vi "Read Pulse driver.vi"(8 "error in (no error)":errorcluster, 11 "Pulse Recorder in":refnum<class "Pulse Recorder Actor.lvclass">) -> (0 "error out":errorcluster, 2 "Pulse Driver.lvclass":refnum<class "Pulse Driver.lvclass">, 3 "Pulse Recorder out":refnum<class "Pulse Recorder Actor.lvclass">)   [LabVIEW 2021, in "Pulse Recorder Actor.lvclass"]
uses:
  Pulse Recorder Actor.lvclass
  Pulse Recorder Actor.lvclass/Pulse Recorder Actor.ctl
  NHMFL_Core/Libraries/Instruments/Pulse Driver/Pulse Driver.lvclass
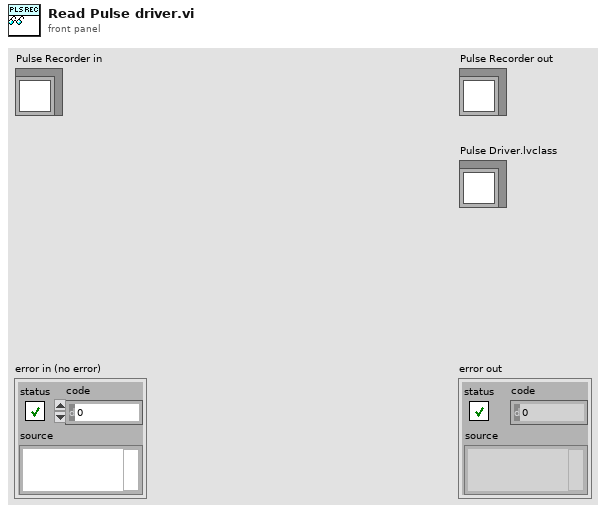
[diagram p1: front panel]
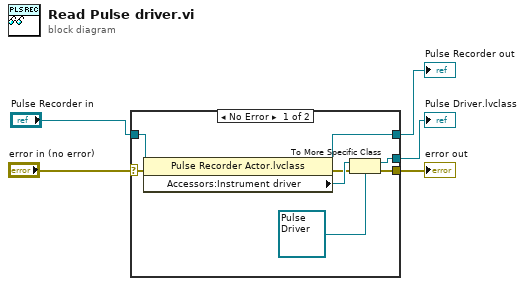
[diagram p0: block diagram]
diagram:
  n1 = case shown="No Error" "error in (no error)" {
    selector: "error in (no error)" -> [w6 w14]
    tunnel: [w7 w14] -> w4
    tunnel: [w12 w15] -> w2
    tunnel: "Pulse Recorder in" -> [w13 w15]
    tunnel: [w10 _] -> w1
    frame No Error {
      n2 = property class="Pulse Recorder Actor.lvclass"(reference=w13, error in=w6) -> (reference out=w12:refnum<class "Pulse Recorder Actor.lvclass">, error out=w8:errorcluster, "Accessors:Instrument driver"=w11:refnum<class "Instrument Driver.lvclass">)
      n3 = To More Specific Class(target class=refnum<class "Pulse Driver.lvclass"> refnum ("Pulse Driver.lvclass"), reference=w11, error in=w8) -> (specific class reference=w10:refnum<class "Pulse Driver.lvclass">, error out=w7:errorcluster)
    }
    frame Error {
    }
  }
  "error out" <- w4
  "Pulse Recorder out" <- w2
  "Pulse Driver.lvclass" <- w1
